vi "Create ByteBuffer.vi"(8 "error in":errorcluster, 10 "default value":u8 format="%02x", 11 "bufSize":i32) -> (0 "error out":errorcluster, 3 "Buffer":refnum<data-value>)   [LabVIEW 2013, in "ByteBuffer.lvclass"]
doc: "This VI creates a ring buffer of set size. This buffer is created in one place in the memory and is then accessed via pointer/reference.\n\nThe Data Type input is required because it defines the place in the memory to correct size thus removing the need for memory reallocation."
uses:
  ByteBuffer.lvclass
  VariantBuffer/VariantBuffer.lvclass
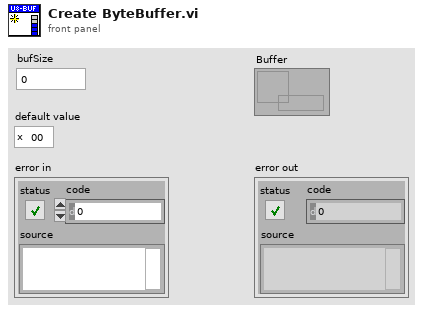
[diagram p1: front panel]
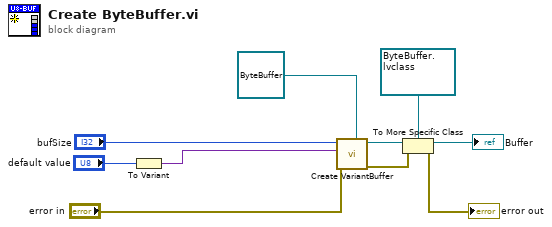
[diagram p0: block diagram]
diagram:
  n1 = To Variant(anything="default value") -> (Variant=w7:variant)
  n2 = call "Create VariantBuffer.vi"("Buffer"=refnum<class "ByteBuffer.lvclass"> refnum ("ByteBuffer.lvclass"), "error in"="error in", "default"=w7, "bufSize"="bufSize") -> ("error out"=w2:errorcluster, "Buffer"=w5:refnum<data-value>)  [unwired: 6 in]
  n3 = To More Specific Class(target class=refnum<data-value> refnum ("Buffer"), reference=w5, error in=w2) -> (specific class reference=→"Buffer":refnum<data-value>, error out=→"error out":errorcluster)
